vi "PH_4_Pos_Selector.draw Knob Pictures.vi"(0 "i ref in":refnum<vi>, 5 "error in":errorcluster) -> (14 "i ref out":refnum<vi>, 17 "Picture Array":picture[](array[picture]), 19 "error out":errorcluster)   [LabVIEW 2014, in "PH_4_Pos_Selector.lvlib"]
uses:
  PH_4_Pos_Selector.lvlib
  CS_Core/CSSystem/CSSystemLib/CSSystemLib.lvlib
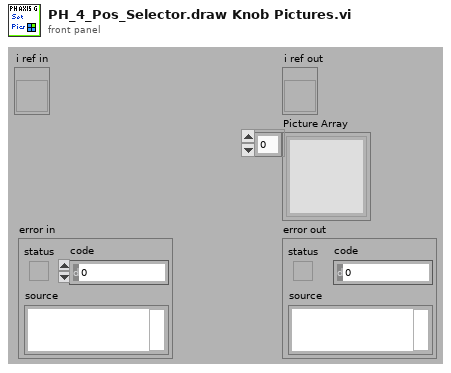
[diagram p1: front panel]
types:
  T1 = typedef "PH_4_Pos_Selector.lvlib/PH_4_Pos_Selector.i attribute.ctl" = cluster{"GUI Refs":cluster{"Position I":refnum<vi>, "Position II":refnum<vi>, "Position III":refnum<vi>, "Position IV":refnum<vi>, "rel. Mode?":refnum<vi>, "Define Selector":refnum<vi>}, "Current Position":T2, "Service ID Position":i32, "Position Array":T3[], "Description Array":string[], "relative Mode":bool, "Wanted Define Selector Position":string}
  T2 = typedef "PH_4_Pos_Selector.lvlib/PH_4_Pos_Selector.Position Selector.ctl" = u16
  T3 = typedef "PH_4_Pos_Selector.lvlib/PH_4_Pos_Selector.Position.ctl" = cluster{"Axis 1":dbl, "Axis 2":dbl}
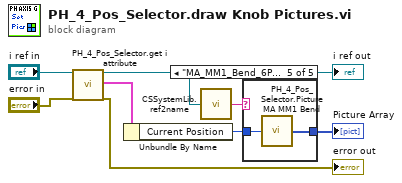
[diagram p0: block diagram]
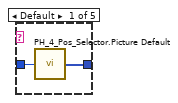
[diagram p2: hidden frame]
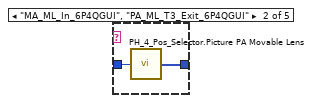
[diagram p3: hidden frame]
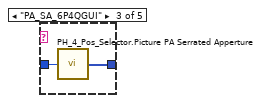
[diagram p4: hidden frame]
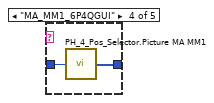
[diagram p5: hidden frame]
diagram:
  n1 = call "PH_4_Pos_Selector.get i attribute.vi"("i ref in"="i ref in", "error in (no error)"="error in") -> ("i ref out"=w4:refnum<vi>, "i attribute"=w5:T1, "error out"=→"error out":errorcluster)  [unwired: 15 in]
  "i ref out" <- w4
  n2 = Unbundle By Name(w5) -> ("Current Position"=w1:T2)
  n3 = call "CSSystemLib.ref2name.vi"("obj refnum"=w4) -> ("name"=w3:string)
  n4 = case shown="\"MA_MM1_Bend_6P4QGUI\"" w3 {
    tunnel: [w10 w12 w14 w15 w17] -> w2
    tunnel: w1 -> [w9 w11 w13 w16 w18]
    frame Default {
      n5 = call "PH_4_Pos_Selector.Picture Default.vi"("Current Position"=w9) -> ("Default Array"=w10:picture[])
    }
    frame "MA_ML_In_6P4QGUI", "PA_ML_T3_Exit_6P4QGUI" {
      n6 = call "PH_4_Pos_Selector.Picture PA Movable Lens.vi"("Current Position"=w11) -> ("Movable Lens Array"=w12:picture[])
    }
    frame "PA_SA_6P4QGUI" {
      n7 = call "PH_4_Pos_Selector.Picture PA Serrated Apperture.vi"("Current Position"=w13) -> ("PA Seratted Apperture Array"=w14:picture[])
    }
    frame "MA_MM1_6P4QGUI" {
      n8 = call "PH_4_Pos_Selector.Picture MA MM1.vi"("State"=w16) -> ("Array MM1"=w15:picture[])
    }
    frame "MA_MM1_Bend_6P4QGUI" {
      n9 = call "PH_4_Pos_Selector.Picture MA MM1 Bend.vi"("State"=w18) -> ("Array MM1 Bend"=w17:picture[])
    }
  }
  "Picture Array" <- w2
